vi "JT_Split_Cluster.vi"(0 "Cluster":T3={"Setpoint - Manual"=0.0, "Rate (K/min)"=0.0, "Activate Tsweep"=FALSE, "Disable Heater"=FALSE, "Update Lakeshores"=FALSE, "Still Heater"=TRUE, "Sorb Heater"=TRUE, "Still Power (mW)"=0.0, "Sorb Power (mW)"=0.0, "V2"=FALSE, "V5"=FALSE, "V1"=FALSE, "V9"=FALSE, "F"=FALSE, "C"=FALSE, "V4"=FALSE, "Dump"=3, "P3"=0.0, "P1"=0.0, "P2"=0.0, "P5"=0.0, "Box Temp"=0.0, "Pressure 1"=0, "Pressure 2"=0, "Pressure 3"=15, "Pressure 4"=13, "Setpoint"=0.0, "MC Heater Output"=0.0, "Still Heater Output"=0.0, "Sorb  Heater Output"=0.0, "Heater"=[], "Pressures"=[]} {"Pressure 4" items=["Time", "LI1CH1", "LI1CH2", "LI2CH1", "LI2CH2", "LI3CH1", "LI3CH2", "Field", "Temperature", "Temperature 2", "Temperatrue 3", "Nitrogen_Level", "Helium_Level", "Heater_LS370", "Sorb_Heater", "Still_Heater", "Capacity", "Loss", "Magnet_Temperature", "Lambda_Pressure", "Lambda_Needle_Valve", "LS370-CH1-T", "LS370-CH2-T", "LS370-CH3-T", "LS370-CH4-T", "LS370-TC-T", "LS370-CH1-R", "LS370-CH2-R", "LS370-CH3-R", "LS370-CH4-R", "LS370-TC-R", "LS372-CH1-T", "LS372-CH2-T", "LS372-CH3-T", "LS372-CH4-T", "LS372-CH5-T", "LS372-CH1-R", "LS372-CH2-R", "LS372-CH3-R", "LS372-CH4-R", "LS372-CH5-R", "Nada", "Keithley_Res", "Keithley_Current", "VTI_Heater", "VTI_Needle Valve", "LS340_Heater", "Keithley_6221_Amplitude", "Keithley_6221_Frequency", "Condense_Pressure", "Still_Pressure", "FP_Out_Pressure", "Dump_Pressure", "V1", "V2", "V4", "V5", "V9", "Forepump", "Compressor", "Keihtley_6221_Offset", "BoxTemp", "By", "Bz", "Phi", "heater-recond (%)", "Dewar Pressure "]; "Pressure 3" items=["Time", "LI1CH1", "LI1CH2", "LI2CH1", "LI2CH2", "LI3CH1", "LI3CH2", "Field", "Temperature", "Temperature 2", "Temperatrue 3", "Nitrogen_Level", "Helium_Level", "Heater_LS370", "Sorb_Heater", "Still_Heater", "Capacity", "Loss", "Magnet_Temperature", "Lambda_Pressure", "Lambda_Needle_Valve", "LS370-CH1-T", "LS370-CH2-T", "LS370-CH3-T", "LS370-CH4-T", "LS370-TC-T", "LS370-CH1-R", "LS370-CH2-R", "LS370-CH3-R", "LS370-CH4-R", "LS370-TC-R", "LS372-CH1-T", "LS372-CH2-T", "LS372-CH3-T", "LS372-CH4-T", "LS372-CH5-T", "LS372-CH1-R", "LS372-CH2-R", "LS372-CH3-R", "LS372-CH4-R", "LS372-CH5-R", "Nada", "Keithley_Res", "Keithley_Current", "VTI_Heater", "VTI_Needle Valve", "LS340_Heater", "Keithley_6221_Amplitude", "Keithley_6221_Frequency", "Condense_Pressure", "Still_Pressure", "FP_Out_Pressure", "Dump_Pressure", "V1", "V2", "V4", "V5", "V9", "Forepump", "Compressor", "Keihtley_6221_Offset", "BoxTemp", "By", "Bz", "Phi", "heater-recond (%)", "Dewar Pressure "]; "Pressure 2" items=["Time", "LI1CH1", "LI1CH2", "LI2CH1", "LI2CH2", "LI3CH1", "LI3CH2", "Field", "Temperature", "Temperature 2", "Temperatrue 3", "Nitrogen_Level", "Helium_Level", "Heater_LS370", "Sorb_Heater", "Still_Heater", "Capacity", "Loss", "Magnet_Temperature", "Lambda_Pressure", "Lambda_Needle_Valve", "LS370-CH1-T", "LS370-CH2-T", "LS370-CH3-T", "LS370-CH4-T", "LS370-TC-T", "LS370-CH1-R", "LS370-CH2-R", "LS370-CH3-R", "LS370-CH4-R", "LS370-TC-R", "LS372-CH1-T", "LS372-CH2-T", "LS372-CH3-T", "LS372-CH4-T", "LS372-CH5-T", "LS372-CH1-R", "LS372-CH2-R", "LS372-CH3-R", "LS372-CH4-R", "LS372-CH5-R", "Nada", "Keithley_Res", "Keithley_Current", "VTI_Heater", "VTI_Needle Valve", "LS340_Heater", "Keithley_6221_Amplitude", "Keithley_6221_Frequency", "Condense_Pressure", "Still_Pressure", "FP_Out_Pressure", "Dump_Pressure", "V1", "V2", "V4", "V5", "V9", "Forepump", "Compressor", "Keihtley_6221_Offset", "BoxTemp", "By", "Bz", "Phi", "heater-recond (%)", "Dewar Pressure "]; "Pressure 1" items=["Time", "LI1CH1", "LI1CH2", "LI2CH1", "LI2CH2", "LI3CH1", "LI3CH2", "Field", "Temperature", "Temperature 2", "Temperatrue 3", "Nitrogen_Level", "Helium_Level", "Heater_LS370", "Sorb_Heater", "Still_Heater", "Capacity", "Loss", "Magnet_Temperature", "Lambda_Pressure", "Lambda_Needle_Valve", "LS370-CH1-T", "LS370-CH2-T", "LS370-CH3-T", "LS370-CH4-T", "LS370-TC-T", "LS370-CH1-R", "LS370-CH2-R", "LS370-CH3-R", "LS370-CH4-R", "LS370-TC-R", "LS372-CH1-T", "LS372-CH2-T", "LS372-CH3-T", "LS372-CH4-T", "LS372-CH5-T", "LS372-CH1-R", "LS372-CH2-R", "LS372-CH3-R", "LS372-CH4-R", "LS372-CH5-R", "Nada", "Keithley_Res", "Keithley_Current", "VTI_Heater", "VTI_Needle Valve", "LS340_Heater", "Keithley_6221_Amplitude", "Keithley_6221_Frequency", "Condense_Pressure", "Still_Pressure", "FP_Out_Pressure", "Dump_Pressure", "V1", "V2", "V4", "V5", "V9", "Forepump", "Compressor", "Keihtley_6221_Offset", "BoxTemp", "By", "Bz", "Phi", "heater-recond (%)", "Dewar Pressure "]; "Dump" scale=0.0..100.0}) -> (1 "Status":T2={"V2"=FALSE, "V5"=FALSE, "V1"=FALSE, "V9"=FALSE, "F"=FALSE, "C"=FALSE, "V4"=FALSE, "Dump"=0, "P3"=0.0, "P1"=3.4572, "P2"=0.0, "P5"=0.0, "Box Temp"=0.0, "Pressure 1"=0, "Pressure 2"=0, "Pressure 3"=15, "Pressure 4"=13, "Setpoint"=0.0, "MC Heater Output"=0.0, "Still Heater Output"=0.0, "Sorb  Heater Output"=0.0, "Heater"=[], "Pressures"=[]} {"Pressure 4" items=["Time", "LI1CH1", "LI1CH2", "LI2CH1", "LI2CH2", "LI3CH1", "LI3CH2", "Field", "Temperature", "Temperature 2", "Temperatrue 3", "Nitrogen_Level", "Helium_Level", "Heater_LS370", "Sorb_Heater", "Still_Heater", "Capacity", "Loss", "Magnet_Temperature", "Lambda_Pressure", "Lambda_Needle_Valve", "LS370-CH1-T", "LS370-CH2-T", "LS370-CH3-T", "LS370-CH4-T", "LS370-TC-T", "LS370-CH1-R", "LS370-CH2-R", "LS370-CH3-R", "LS370-CH4-R", "LS370-TC-R", "LS372-CH1-T", "LS372-CH2-T", "LS372-CH3-T", "LS372-CH4-T", "LS372-CH5-T", "LS372-CH1-R", "LS372-CH2-R", "LS372-CH3-R", "LS372-CH4-R", "LS372-CH5-R", "Nada", "Keithley_Res", "Keithley_Current", "VTI_Heater", "VTI_Needle Valve", "LS340_Heater", "Keithley_6221_Amplitude", "Keithley_6221_Frequency", "Condense_Pressure", "Still_Pressure", "FP_Out_Pressure", "Dump_Pressure", "V1", "V2", "V4", "V5", "V9", "Forepump", "Compressor", "Keihtley_6221_Offset", "BoxTemp", "By", "Bz", "Phi", "heater-recond (%)", "Dewar Pressure "]; "Pressure 3" items=["Time", "LI1CH1", "LI1CH2", "LI2CH1", "LI2CH2", "LI3CH1", "LI3CH2", "Field", "Temperature", "Temperature 2", "Temperatrue 3", "Nitrogen_Level", "Helium_Level", "Heater_LS370", "Sorb_Heater", "Still_Heater", "Capacity", "Loss", "Magnet_Temperature", "Lambda_Pressure", "Lambda_Needle_Valve", "LS370-CH1-T", "LS370-CH2-T", "LS370-CH3-T", "LS370-CH4-T", "LS370-TC-T", "LS370-CH1-R", "LS370-CH2-R", "LS370-CH3-R", "LS370-CH4-R", "LS370-TC-R", "LS372-CH1-T", "LS372-CH2-T", "LS372-CH3-T", "LS372-CH4-T", "LS372-CH5-T", "LS372-CH1-R", "LS372-CH2-R", "LS372-CH3-R", "LS372-CH4-R", "LS372-CH5-R", "Nada", "Keithley_Res", "Keithley_Current", "VTI_Heater", "VTI_Needle Valve", "LS340_Heater", "Keithley_6221_Amplitude", "Keithley_6221_Frequency", "Condense_Pressure", "Still_Pressure", "FP_Out_Pressure", "Dump_Pressure", "V1", "V2", "V4", "V5", "V9", "Forepump", "Compressor", "Keihtley_6221_Offset", "BoxTemp", "By", "Bz", "Phi", "heater-recond (%)", "Dewar Pressure "]; "Pressure 2" items=["Time", "LI1CH1", "LI1CH2", "LI2CH1", "LI2CH2", "LI3CH1", "LI3CH2", "Field", "Temperature", "Temperature 2", "Temperatrue 3", "Nitrogen_Level", "Helium_Level", "Heater_LS370", "Sorb_Heater", "Still_Heater", "Capacity", "Loss", "Magnet_Temperature", "Lambda_Pressure", "Lambda_Needle_Valve", "LS370-CH1-T", "LS370-CH2-T", "LS370-CH3-T", "LS370-CH4-T", "LS370-TC-T", "LS370-CH1-R", "LS370-CH2-R", "LS370-CH3-R", "LS370-CH4-R", "LS370-TC-R", "LS372-CH1-T", "LS372-CH2-T", "LS372-CH3-T", "LS372-CH4-T", "LS372-CH5-T", "LS372-CH1-R", "LS372-CH2-R", "LS372-CH3-R", "LS372-CH4-R", "LS372-CH5-R", "Nada", "Keithley_Res", "Keithley_Current", "VTI_Heater", "VTI_Needle Valve", "LS340_Heater", "Keithley_6221_Amplitude", "Keithley_6221_Frequency", "Condense_Pressure", "Still_Pressure", "FP_Out_Pressure", "Dump_Pressure", "V1", "V2", "V4", "V5", "V9", "Forepump", "Compressor", "Keihtley_6221_Offset", "BoxTemp", "By", "Bz", "Phi", "heater-recond (%)", "Dewar Pressure "]; "Pressure 1" items=["Time", "LI1CH1", "LI1CH2", "LI2CH1", "LI2CH2", "LI3CH1", "LI3CH2", "Field", "Temperature", "Temperature 2", "Temperatrue 3", "Nitrogen_Level", "Helium_Level", "Heater_LS370", "Sorb_Heater", "Still_Heater", "Capacity", "Loss", "Magnet_Temperature", "Lambda_Pressure", "Lambda_Needle_Valve", "LS370-CH1-T", "LS370-CH2-T", "LS370-CH3-T", "LS370-CH4-T", "LS370-TC-T", "LS370-CH1-R", "LS370-CH2-R", "LS370-CH3-R", "LS370-CH4-R", "LS370-TC-R", "LS372-CH1-T", "LS372-CH2-T", "LS372-CH3-T", "LS372-CH4-T", "LS372-CH5-T", "LS372-CH1-R", "LS372-CH2-R", "LS372-CH3-R", "LS372-CH4-R", "LS372-CH5-R", "Nada", "Keithley_Res", "Keithley_Current", "VTI_Heater", "VTI_Needle Valve", "LS340_Heater", "Keithley_6221_Amplitude", "Keithley_6221_Frequency", "Condense_Pressure", "Still_Pressure", "FP_Out_Pressure", "Dump_Pressure", "V1", "V2", "V4", "V5", "V9", "Forepump", "Compressor", "Keihtley_6221_Offset", "BoxTemp", "By", "Bz", "Phi", "heater-recond (%)", "Dewar Pressure "]; "Dump" scale=0.0..100.0}, 2 "Control":T1={"Disable Heater"=FALSE, "Activate Tsweep"=FALSE, "Update Lakeshores"=FALSE, "Setpoint - Manual"=0.0, "Rate (K/min)"=0.0, "Sorb Power (mW)"=3.4572, "Still Power (mW)"=0.0, "Sorb Heater"=FALSE, "Still Heater"=FALSE, "Set Temperature Sweep Main"=FALSE})   [LabVIEW 2016]
uses:
  JT/JT-Cluster.ctl
  JT/JT-Status.ctl
  LS370/LS370-Control.ctl
panel:
  # "Dill. unit"
  # "LN2\nTrap"
  # "12"
  # "15"
  # "Dill. unit"
  # "LN2\nTrap"
  # "12"
  # "15"
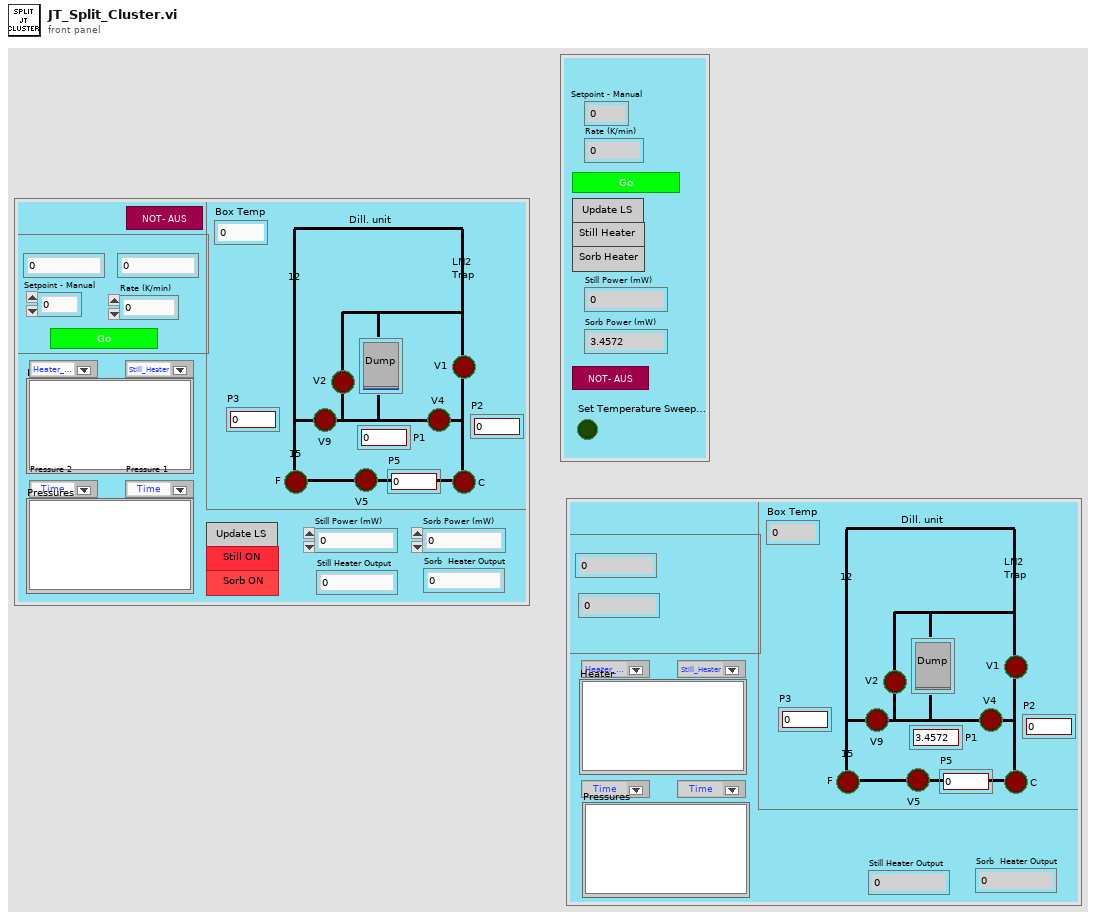
[diagram p1: front panel]
types:
  T1 = typedef "LS370-Control.ctl" = cluster{"Disable Heater":bool, "Activate Tsweep":bool, "Update Lakeshores":bool, "Setpoint - Manual":dbl, "Rate (K/min)":dbl, "Sorb Power (mW)":dbl, "Still Power (mW)":dbl, "Sorb Heater":bool, "Still Heater":bool, "Set Temperature Sweep Main":bool}
  T2 = typedef "JT-Status.ctl" = cluster{"V2":bool, "V5":bool, "V1":bool, "V9":bool, "F":bool, "C":bool, "V4":bool, "Dump":u8, "P3":dbl, "P1":dbl, "P2":dbl, "P5":dbl, "Box Temp":dbl, "Pressure 1":i16, "Pressure 2":i16, "Pressure 3":i16, "Pressure 4":i16, "Setpoint":dbl, "MC Heater Output":dbl, "Still Heater Output":dbl, "Sorb  Heater Output":dbl, "Heater":dbl[][], "Pressures":dbl[][]}
  T3 = typedef "JT-Cluster.ctl" = cluster{"Setpoint - Manual":dbl, "Rate (K/min)":dbl, "Activate Tsweep":bool, "Disable Heater":bool, "Update Lakeshores":bool, "Still Heater":bool, "Sorb Heater":bool, "Still Power (mW)":dbl, "Sorb Power (mW)":dbl, "V2":bool, "V5":bool, "V1":bool, "V9":bool, "F":bool, "C":bool, "V4":bool, "Dump":u8, "P3":dbl, "P1":dbl, "P2":dbl, "P5":dbl, "Box Temp":dbl, "Pressure 1":i16, "Pressure 2":i16, "Pressure 3":i16, "Pressure 4":i16, "Setpoint":dbl, "MC Heater Output":dbl, "Still Heater Output":dbl, "Sorb  Heater Output":dbl, "Heater":dbl[][], "Pressures":dbl[][]}
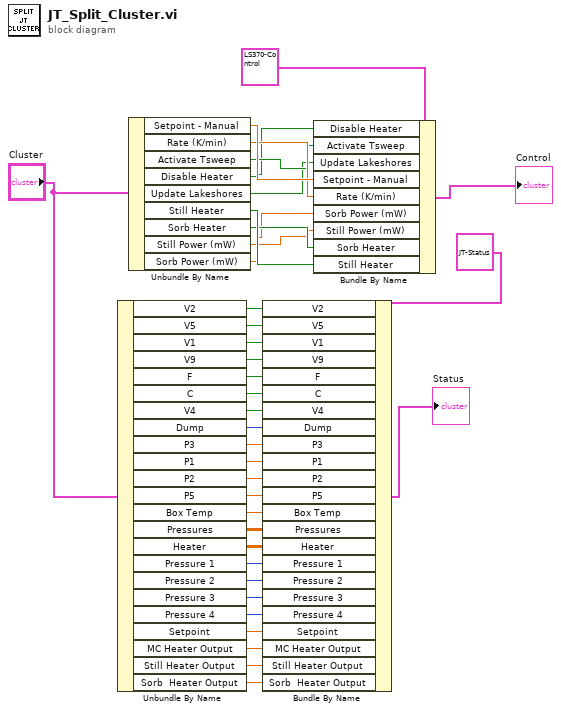
[diagram p0: block diagram]
diagram:
  n1 = Unbundle By Name("Cluster") -> ("V2"=w24:bool, "V5"=w23:bool, "V1"=w22:bool, "V9"=w21:bool, "F"=w20:bool, "C"=w19:bool, "V4"=w18:bool, "Dump"=w17:u8, "P3"=w15:dbl, "P1"=w16:dbl, "P2"=w14:dbl, "P5"=w13:dbl, "Box Temp"=w12:dbl, "Pressures"=w2:dbl[][], "Heater"=w1:dbl[][], "Pressure 1"=w11:i16, "Pressure 2"=w10:i16, "Pressure 3"=w9:i16, "Pressure 4"=w8:i16, "Setpoint"=w7:dbl, "MC Heater Output"=w6:dbl, "Still Heater Output"=w5:dbl, "Sorb  Heater Output"=w4:dbl)
  n2 = Unbundle By Name("Cluster") -> ("Setpoint - Manual"=w35:dbl, "Rate (K/min)"=w34:dbl, "Activate Tsweep"=w33:bool, "Disable Heater"=w32:bool, "Update Lakeshores"=w31:bool, "Still Heater"=w30:bool, "Sorb Heater"=w29:bool, "Still Power (mW)"=w28:dbl, "Sorb Power (mW)"=w27:dbl)
  n3 = Bundle By Name(cluster=T2 {"V2"=FALSE, "V5"=FALSE, "V1"=FALSE, "V9"=FALSE, "F"=FALSE, "C"=FALSE, "V4"=FALSE, "Dump"=0, "P3"=0.0, "P1"=3.4572, "P2"=0.0, "P5"=0.0, "Box Temp"=0.0, "Pressure 1"=0, "Pressure 2"=0, "Pressure 3"=15, "Pressure 4"=13, "Setpoint"=0.0, "MC Heater Output"=0.0, "Still Heater Output"=0.0, "Sorb  Heater Output"=0.0, "Heater"=[], "Pressures"=[]} ("Status 2"), "V2"=w24, "V5"=w23, "V1"=w22, "V9"=w21, "F"=w20, "C"=w19, "V4"=w18, "Dump"=w17, "P3"=w15, "P1"=w16, "P2"=w14, "P5"=w13, "Box Temp"=w12, "Pressures"=w2, "Heater"=w1, "Pressure 1"=w11, "Pressure 2"=w10, "Pressure 3"=w9, "Pressure 4"=w8, "Setpoint"=w7, "MC Heater Output"=w6, "Still Heater Output"=w5, "Sorb  Heater Output"=w4) -> (→"Status":T2)
  n4 = Bundle By Name(cluster=T1 {"Disable Heater"=FALSE, "Activate Tsweep"=FALSE, "Update Lakeshores"=FALSE, "Setpoint - Manual"=0.0, "Rate (K/min)"=0.0, "Sorb Power (mW)"=3.4572, "Still Power (mW)"=0.0, "Sorb Heater"=FALSE, "Still Heater"=FALSE, "Set Temperature Sweep Main"=FALSE} ("JT-Cluster"), "Disable Heater"=w32, "Activate Tsweep"=w33, "Update Lakeshores"=w31, "Setpoint - Manual"=w35, "Rate (K/min)"=w34, "Sorb Power (mW)"=w27, "Still Power (mW)"=w28, "Sorb Heater"=w29, "Still Heater"=w30) -> (→"Control":T1)
